vi "Get Module Execution Status by ref.vi"(11 "Vi Ref":refnum<vi>) -> (0 "error out":errorcluster, 2 "Status":string)   [LabVIEW 2020, in "DQMH_API.lvlib"]
doc: "This VI checks the Main.vi State of the selected DQMH Module"
uses:
  DQMH_API.lvlib
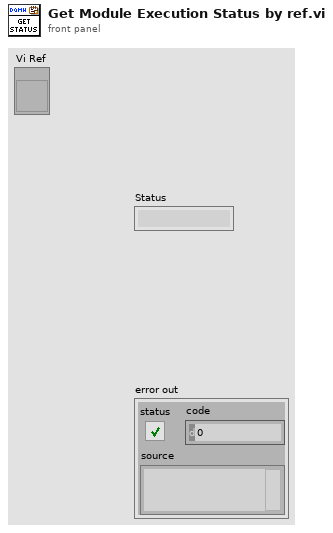
[diagram p1: front panel]
types:
  T1 = enum32{"Bad", "Idle", "Run top level", "Running"}
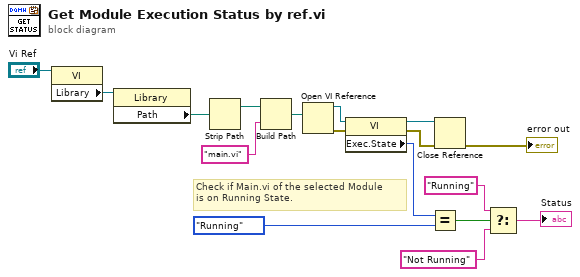
[diagram p0: block diagram]
diagram:
  # "Check if Main.vi of the selected Module\nis on Running State."
  n1 = property class="VI"(reference="Vi Ref") -> ("Library"=w1:refnum<vi>)  [unwired: 1 in, 2 out]
  n2 = property class="Library"(reference=w1) -> ("Path"=w14:path)  [unwired: 1 in, 2 out]
  n3 = Strip Path(path=w14) -> (stripped path=w13:path)  [unwired: 1 out]
  n4 = Build Path(base path=w13, name or relative path="main.vi" ("string")) -> (appended path=w11:path)
  n5 = Open VI Reference(vi path=w11) -> (vi reference=w10:refnum<vi>, error out=w15:errorcluster)  [unwired: 5 in]
  n6 = property class="VI"(reference=w10, error in=w15) -> (reference out=w7:refnum<vi>, error out=w16:errorcluster, "Exec.State"=w9:T1)
  n7 = Equal?(x=w9, y=T1."Running") -> (x = y?=w4:bool)
  n8 = Close Reference(reference=w7, error in (no error)=w16) -> (error out=→"error out":errorcluster)
  n9 = Select(t="Running", s=w4, f="Not Running") -> (s? t:f=→"Status":string)
